vi "DataAcqMasterHD.vi"(0 "Avg Num":i32=1, 1 "2-D motor":bool, 2 "Type of scan":u16, 3 "Move motor":bool, 4 "Compile":bool, 5 "Therapy (T)":bool, 7 "Xmit Ring":i16, 9 "Current Plane":i32, 10 "lines per plane mod":i32, 11 "Total steps in line":i32, 12 "Acqiris ID":u32, 13 "Reverse ?":bool, 15 "CTR1":bool, 16 "start value":dbl, 17 "Motion System":u16, 18 "scan axis":i32, 19 "Motion Bd ID":T1 min=1 max=32 step=1) -> (20 "Samples Returned":i32, 21 "Motion error":bool, 22 "Timeout":bool, 23 "Raw VGain (scale)":dbl, 24 "Atts":dbl[](array[numeric]), 25 "Stacked Data":i16[][][](array[numeric]), 26 "error out":errorcluster)   [LabVIEW 2022 SP3]
uses:
  Motion Controllers/-MotionRoutines/MotionGlobals.vi
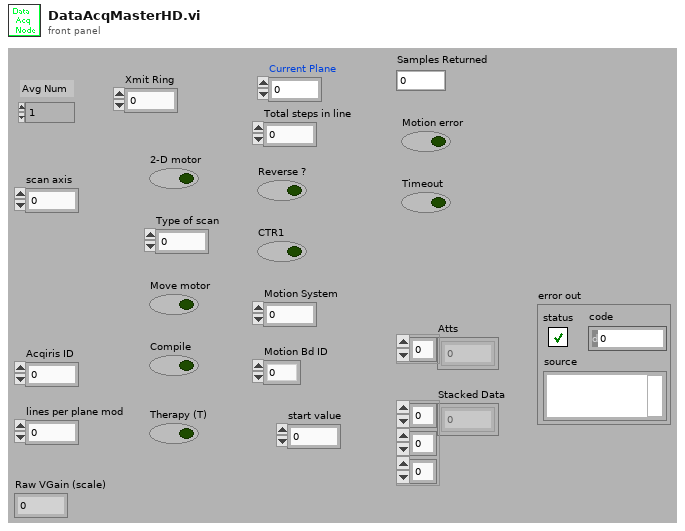
[diagram p1: front panel]
types:
  T1 = typedef "Board Id" = u8
  T2 = typedef "location.ctl" = enum16{"Automatic", "WCM Main", "Hawaii", "Columbia MM3000", "Columbia  NI System", "NYU", "RRI 2", "UHI Allen", "CUMC RT", "Chiba", "Stony Brook", "WCM Microscopy", "WCM Aeoretch", "WCM Optics Lab", "WCM Main 2Axis", "WCM Rotation", "WCM SAM SMAC", "SERI GP"}
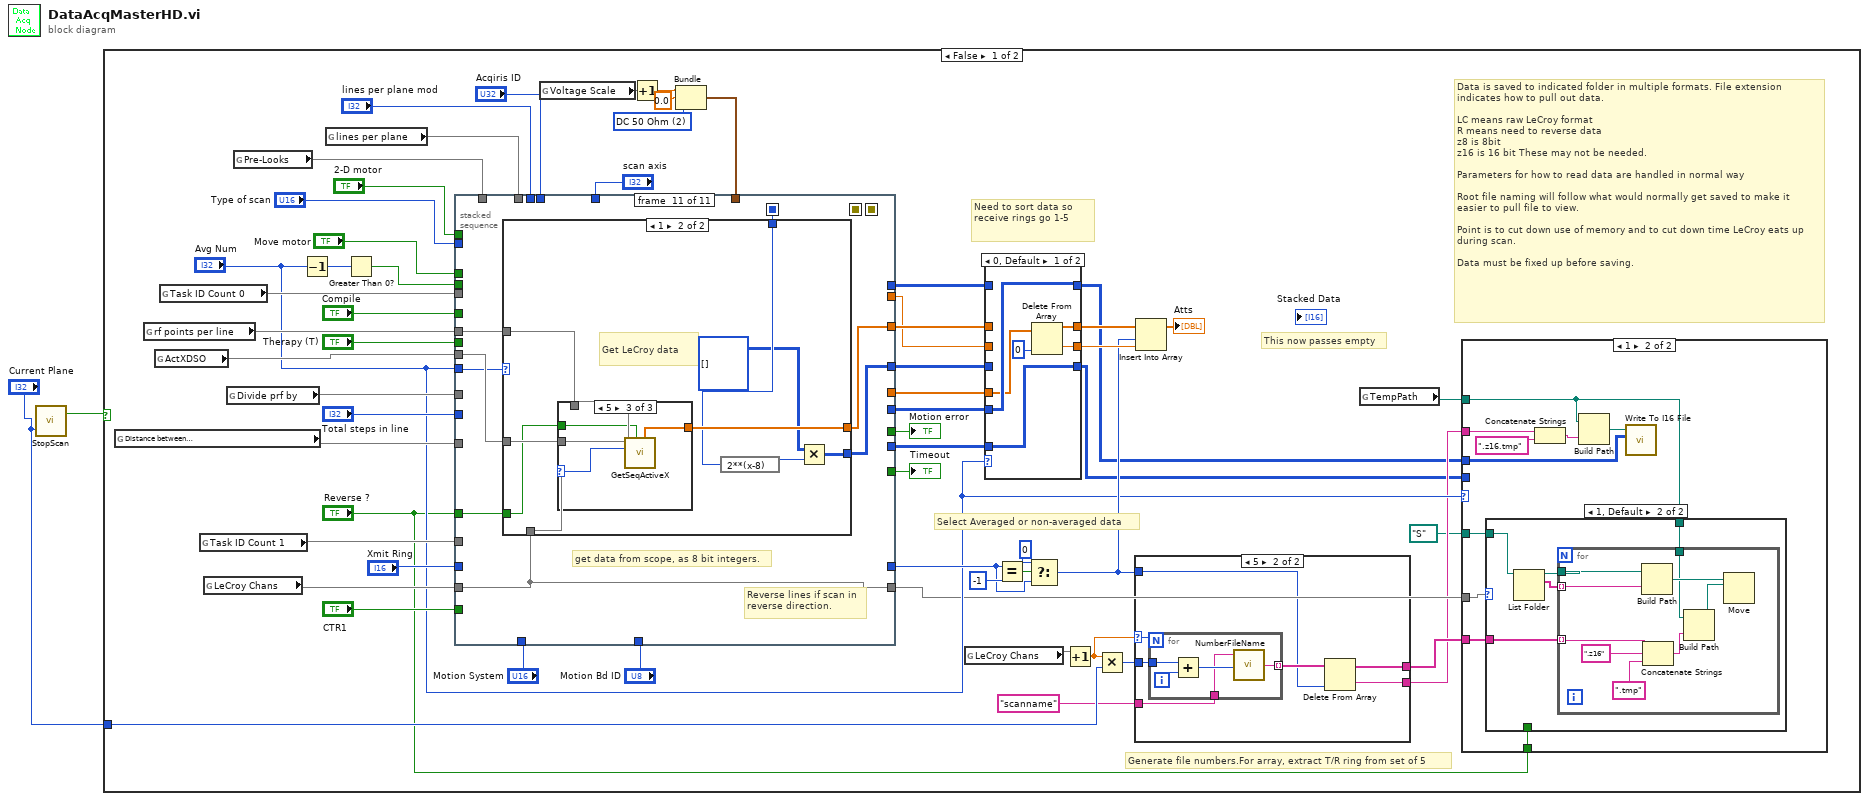
[diagram p0: block diagram]
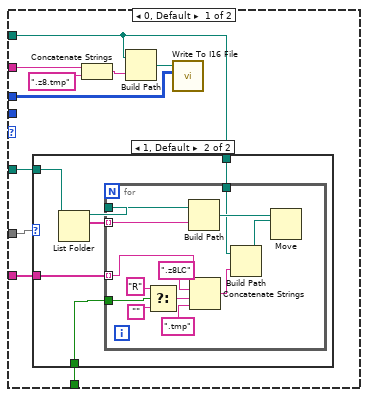
[diagram p2: hidden frame]
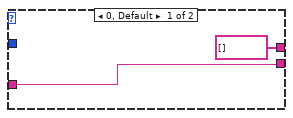
[diagram p5: hidden frame]
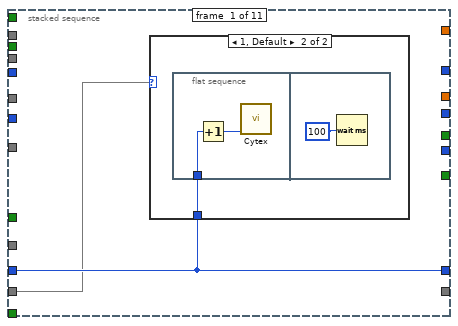
[diagram p7: hidden frame]
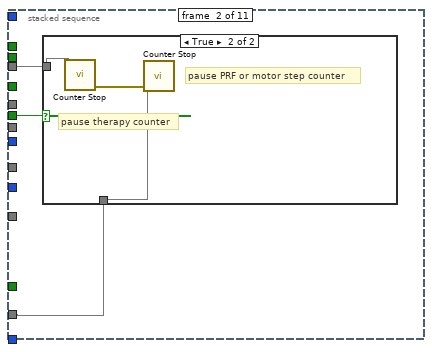
[diagram p9: hidden frame]
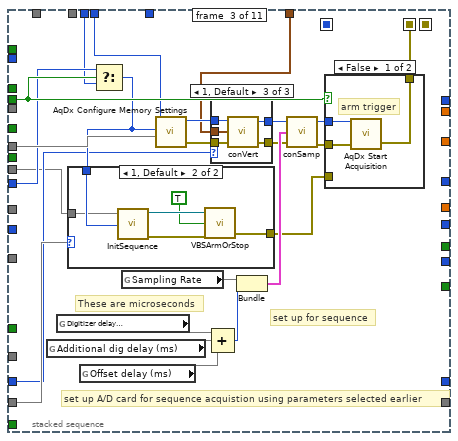
[diagram p11: hidden frame]
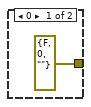
[diagram p15: hidden frame]
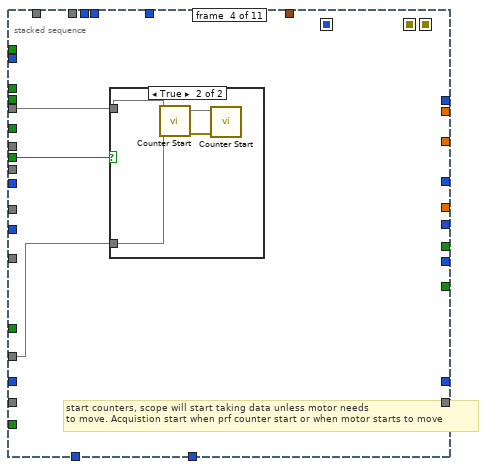
[diagram p16: hidden frame]
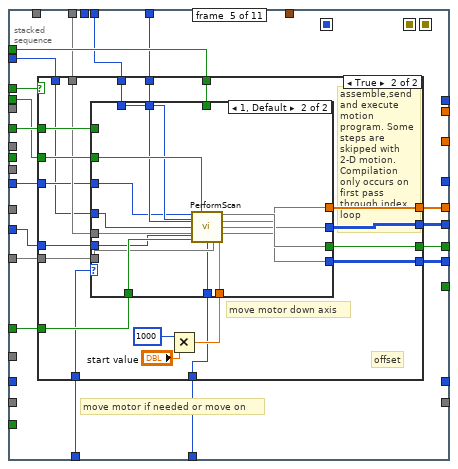
[diagram p18: hidden frame]
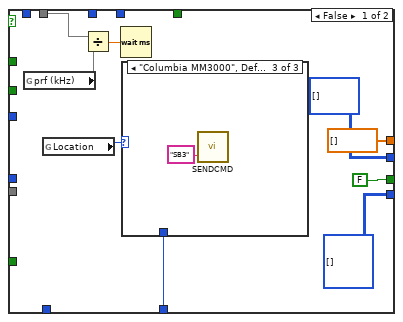
[diagram p19: hidden frame]
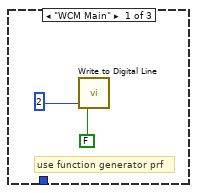
[diagram p20: hidden frame]
diagram:
  n1 = call "StopScan.vi"("Current Plane"="Current Plane") -> ("Stop Now? Dup"=w2:bool)  [unwired: 2 in]
  n2 = case shown="False" w2 {
    tunnel: "Current Plane" -> [w17 _]
    frame False {
      w24 = u16 2 items=["DC 1 MOhm", "AC 1 MOhm", "DC 50 Ohm", "AC 50 OHM"] ("Coupling")
      # "This now passes empty"
      # "Data is saved to indicated folder in multiple formats. File extension indicates how to pull out data.\n\nLC means raw LeCroy format\nR means need to reverse data\nz8 is 8bit\nz16 is 16 bit These may not be needed.\n\nParameters for how to read data are handled in normal way\n\nRoot file naming will follow what would normally get saved to make it easier to pull file to view.\n\nPoint is to cut down use of memory and to cut down time LeCroy eats up during scan.\n\nData must be fixed up before saving."
      # "Generate file numbers.For array, extract T/R ring from set of 5"
      # "Need to sort data so receive rings go 1-5"
      # "Select Averaged or non-averaged data"
      n3 = global read "MotionGlobals.vi" "Distance between\nscan lines (mm)"() -> (w49)
      n4 = global read "MotionGlobals.vi" "rf points per line"() -> (w48)
      n5 = global read "MotionGlobals.vi" "ActXDSO"() -> (w18)
      n6 = global read "MotionGlobals.vi" "Task ID Count 0"() -> (w22)
      n7 = global read "MotionGlobals.vi" "Task ID Count 1"() -> (w21)
      n8 = global read "MotionGlobals.vi" "LeCroy Chans"() -> (w44)
      n9 = global read "MotionGlobals.vi" "Divide prf by"() -> (w45)
      n10 = global read "MotionGlobals.vi" "Pre-Looks"() -> (w46)
      n11 = Decrement(x="Avg Num") -> (x-1=w19:i32)
      n12 = global read "MotionGlobals.vi" "lines per plane"() -> (w47)
      n13 = Greater Than 0?(x=w19) -> (x > 0?=w20:bool)
      n14 = global read "MotionGlobals.vi" "Voltage Scale"() -> (w25)
      n15 = Increment(x=w25) -> (x+1=w26:dbl)
      n16 = Bundle(w26, "Offset"=0.0, "Coupling"=w24) -> (w23:cluster{dbl, "Offset":dbl, "Coupling":u16})  [unwired: 1 in]
      n17 = stacked-sequence {
        seq-local: [_ _ w168 _ _ _ _ _ _ _ _] -> [_ _ _ _ _ w289 _ _ _ _ _]
        seq-local: [_ _ _ _ _ w287 _ _ _ _ _] -> [_ _ _ _ _ _ _ _ w340 _ _]
        seq-local: [_ _ _ _ _ _ _ _ w334 _ _] -> [_ _ _ _ _ _ _ _ _ _ w371]
        tunnel: "Therapy (T)" -> [_ w147 _ w196 _ _ w320 _ _ _ _]
        tunnel: w45 -> [_ _ _ _ _ _ _ _ w342 _ _]
        tunnel: "Move motor" -> [_ _ _ _ w219 _ _ w326 _ _ _]
        tunnel: "2-D motor" -> [_ _ _ _ w217 _ _ _ _ _ _]
        tunnel: "scan axis" -> [_ _ _ _ w213 _ _ _ _ _ _]
        tunnel: "Reverse ?" -> [_ _ _ _ w218 _ _ _ w338 _ w378]
        tunnel: "lines per plane mod" -> [_ _ w154 _ _ _ _ _ _ _ _]
        tunnel: "Total steps in line" -> [_ _ _ _ w215 _ _ _ _ _ _]
        tunnel: "Compile" -> [_ _ _ _ w216 _ _ _ _ _ _]
        tunnel: "CTR1" -> [_ _ _ _ _ _ _ _ _ _ _]
        tunnel: [_ _ _ _ _ w288 _ _ _ _ _] -> w57
        tunnel: "Acqiris ID" -> [_ _ w156 _ w208 w290 _ _ w339 _ _]
        tunnel: [_ _ _ _ _ _ _ _ w345 _ _] -> w42
        tunnel: "Type of scan" -> [_ _ _ _ w202 _ _ _ w344 _ _]
        tunnel: w47 -> [_ _ _ _ w214 w285 _ _ w343 _ _]
        tunnel: w46 -> [_ _ _ _ _ _ _ _ w341 _ _]
        tunnel: [_ _ _ _ w212 _ _ _ _ _ _] -> w60
        tunnel: "Motion System" -> [_ _ _ _ w211 _ _ _ _ _ _]
        tunnel: "Motion Bd ID" -> [_ _ _ _ w210 _ _ w325 _ _ _]
        tunnel: [_ _ _ _ _ _ _ _ _ _ w373] -> w40
        tunnel: w21 -> [_ w146 _ w197 _ _ w319 _ _ _ _]
        tunnel: w22 -> [_ w148 _ w198 _ _ w321 _ _ _ _]
        tunnel: w18 -> [_ _ w153 _ _ _ _ _ _ w365 w377]
        tunnel: w49 -> [_ _ _ _ w209 _ _ _ _ _ _]
        tunnel: w44 -> [w140 _ w163 _ _ _ _ _ _ w363 w374]
        tunnel: w48 -> [_ _ w165 _ _ _ _ _ w337 _ w376]
        tunnel: w20 -> [_ _ w166 _ w207 _ _ _ _ _ _]
        tunnel: "Avg Num" -> [_ _ w155 _ w206 w286 _ _ w336 w364 w375]
        tunnel: [_ _ _ _ w205 _ _ _ _ _ _] -> w39
        tunnel: [_ _ _ _ w204 _ _ _ _ _ _] -> w37
        tunnel: [_ _ _ _ w203 _ _ _ _ _ _] -> w38
        tunnel: [_ _ _ _ _ _ _ _ _ _ w372] -> w41
        tunnel: [w141 _ _ _ _ _ _ _ _ _ _] -> w29
        tunnel: "Xmit Ring" -> [w141 _ w158 _ _ _ _ _ _ _ _]
        tunnel: [_ _ _ _ _ _ _ _ w335 _ _] -> w32
        tunnel: w23 -> [_ _ w157 _ _ _ _ _ _ _ _]
        tunnel: [_ _ _ _ _ _ _ _ _ _ w374] -> w10
        frame #0 {
          n18 = case shown="1, Default" w140 {
            tunnel: w141 -> [_ w142]
            frame 0 {
            }
            frame 1, Default {
              n19 = flat-sequence {
                tunnel: w142 -> [w144]
                frame #0 {
                  n20 = Increment(x=w144) -> (x+1=w143:i16)
                  n21 = call "Cytex.vi"("Xmit Ring"=w143) -> ()  [unwired: 1 in, 2 out]
                }
                frame #1 {
                  n22 = Wait (ms)(milliseconds to wait=100) -> ()  [unwired: 1 out]
                }
              }
            }
          }
        }
        frame #1 {
          n23 = case shown="True" w147 {
            tunnel: w148 -> [_ w151]
            tunnel: w146 -> [_ w149]
            frame False {
            }
            frame True {
              # "pause PRF or motor step counter"
              # "pause therapy counter"
              n24 = call <vilib>:"Counter Stop.vi"("taskID"=w151) -> ("error out"=w150:errorcluster)  [unwired: 5 in, 1 out]
              n25 = call <vilib>:"Counter Stop.vi"("error in (no error)"=w150, "taskID"=w149) -> ()  [unwired: 4 in, 2 out]
            }
          }
        }
        frame #2 {
          # "These are microseconds"
          # "set up for sequence"
          # "set up A/D card for sequence acquistion using parameters selected earlier"
          n26 = global read "MotionGlobals.vi" "Additional dig delay (ms)"() -> (w171)
          n27 = global read "MotionGlobals.vi" "Digitizer delay\n (ms)"() -> (w174)
          n28 = global read "MotionGlobals.vi" "Offset delay (ms)"() -> (w167)
          n29 = Select(t=w155, s=w166, f=w154) -> (s? t:f=w164:i32)
          n30 = case shown="1, Default" w163 {
            tunnel: w164 -> [_ w195]
            tunnel: w153 -> [_ w194]
            tunnel: [errorcluster {"status"=FALSE, "code"=0, "source"=""} ("error out") w190] -> w152
            frame 0 {
            }
            frame 1, Default {
              n31 = call "InitSequence.vi"("ActXDSO In"=w194, "Num of Sequences"=w195) -> ("ActXDSO Out"=w193:refnum<k7>, "error out"=w192:errorcluster)  [unwired: 5 in]
              n32 = call "VBSArmOrStop.vi"("error in (no error)"=w192, "Arm T/Stop F"=TRUE, "ActXDSO In"=w193) -> ("error out"=w190:errorcluster)  [unwired: 1 in, 1 out]
            }
          }
          n33 = global read "MotionGlobals.vi" "Sampling Rate"() -> (w173)
          n34 = call "AqDx Configure Memory Settings.vi"("Number of Samples (1000)"=w165, "Number of Segments (1)"=w164, "Instrument ID"=w156) -> ("error out"=w159:errorcluster, "dup Instrument ID"=w160:u32)  [unwired: 3 in]
          n35 = case shown="1, Default" w158 {
            tunnel: [w177 w179 w184] -> w162
            tunnel: [w176 w178 w183] -> w161
            tunnel: w160 -> [w177 w179 w182]
            tunnel: w159 -> [w176 w178 w181]
            tunnel: w157 -> [_ _ w180]
            frame 0 {
            }
            frame -1 {
            }
            frame 1, Default {
              n36 = call "conVert.vi"("InstrumentID"=w182, "V scale"=w180, "error in"=w181) -> ("Status"=w184:i32, "error out"=w183:errorcluster)  [unwired: 3 in]
            }
          }
          n37 = Compound Arithmetic op=ADD(w174, w171, w167) -> (w172:i32)
          n38 = Bundle("Sampling Rate"=w173, w172) -> (w175:cluster{"Sampling Rate":void, i32})  [unwired: 1 in]
          n39 = call "conSamp.vi"("error in"=w161, "Sampling"=w175, "InstrumentID"=w162) -> ("error out"=w169:errorcluster, "DUP ID"=w170:u32)
          n40 = case shown="False" w166 {
            tunnel: w170 -> [w187 _]
            tunnel: w169 -> [w186 w188]
            tunnel: [w185 w188] -> w168
            tunnel: w152 -> [_ _]
            frame False {
              # "arm trigger"
              n41 = call "AqDx Start Acquisition.vi"("error in (no error)"=w186, "Instrument ID"=w187) -> ("error out"=w185:errorcluster)  [unwired: 1 in, 1 out]
            }
            frame True {
            }
          }
        }
        frame #3 {
          # "start counters, scope will start taking data unless motor needs\nto move. Acquistion start when prf counter start or when motor starts to move"
          n42 = case shown="True" w196 {
            tunnel: w198 -> [_ w201]
            tunnel: w197 -> [_ w199]
            frame False {
            }
            frame True {
              n43 = call <vilib>:"Counter Start.vi"("taskID"=w201) -> ("error out"=w200:errorcluster)  [unwired: 9 in, 1 out]
              n44 = call <vilib>:"Counter Start.vi"("error in (no error)"=w200, "taskID"=w199) -> ()  [unwired: 8 in, 2 out]
            }
          }
        }
        frame #4 {
          # "move motor if needed or move on"
          n45 = case shown="True" w219 {
            tunnel: w209 -> [_ w251]
            tunnel: w218 -> [_ w253]
            tunnel: w207 -> [_ w252]
            tunnel: w217 -> [_ w250]
            tunnel: w216 -> [_ w249]
            tunnel: w215 -> [_ w248]
            tunnel: w214 -> [w221 w244]
            tunnel: w213 -> [_ w247]
            tunnel: [FALSE w246] -> w212
            tunnel: w211 -> [_ w245]
            tunnel: w210 -> [w226 w235]
            tunnel: w208 -> [_ w243]
            tunnel: w206 -> [_ w242]
            tunnel: [dbl[] [] ("Att (dB)") w241] -> w205
            tunnel: [i16[][] [] ("Acqiris Avg") w240] -> w204
            tunnel: [i16[][][] [] ("Acqiris Avg") w239] -> w203
            tunnel: w202 -> [_ w234]
            frame False {
              n46 = global read "MotionGlobals.vi" "prf (kHz)"() -> (w220)
              n47 = global read "MotionGlobals.vi" "Location"() -> (w227:T2)
              n48 = Divide(x=w221, y=w220) -> (x/y=w222:dbl)
              n49 = Wait (ms)(milliseconds to wait=w222) -> ()  [unwired: 1 out]
              n50 = case shown="\"Columbia MM3000\", Default" w227 {
                tunnel: w226 -> [_ w231 _]
                frame "WCM Main" {
                  # "use function generator prf"
                  n51 = call <vilib>:"Write to Digital Line.vi"("line"=2, "line state"=FALSE) -> ()  [unwired: 7 in]
                }
                frame "Hawaii" {
                  # "Use BreakPt PRF"
                  n52 = call <vilib>:"Run Program.flx"("Program (1)"=3, "Board ID"=w231) -> ()  [unwired: 4 in, 3 out]
                }
                frame "Columbia MM3000", Default {
                  n53 = call "SENDCMD.VI"("MM2000 Command (ASCII String)"="SB3") -> ()  [unwired: 2 in, 1 out]
                }
              }
            }
            frame True {
              # "assemble,send and execute\nmotion program. Some steps are\nskipped with 2-D motion. Compilation only occurs on first pass through index loop"
              # "offset"
              # "move motor down axis"
              n54 = Multiply(x=1000, y="start value") -> (x*y=w236:dbl)
              n55 = case shown="1, Default" w245 {
                tunnel: w253 -> [w269 w284]
                tunnel: w252 -> [w268 w283]
                tunnel: w251 -> [w267 w282]
                tunnel: w250 -> [w266 _]
                tunnel: w249 -> [w265 _]
                tunnel: w248 -> [w264 w281]
                tunnel: w247 -> [w263 w280]
                tunnel: [w256 w276] -> w246
                tunnel: w244 -> [w262 w279]
                tunnel: w243 -> [w261 w278]
                tunnel: w242 -> [w260 w277]
                tunnel: [w259 w273] -> w241
                tunnel: [w258 w274] -> w240
                tunnel: [w257 w275] -> w239
                tunnel: w236 -> [w255 w272]
                tunnel: w235 -> [_ w271]
                tunnel: w234 -> [w254 w270]
                frame 0 {
                  n56 = call "SendProgram.vi"("Type of scan"=w254, "Line Axis"=w263, "Avg Num"=w260, "lines per scan plane"=w262, "Reverse ?"=w269, "Therapy/AVG ?"=w268, 7:w264, 8:w261, 12:w266, 13:w267, 14:w265, "Offset"=w255) -> ("Error Status"=w256:bool, 16:w259, 17:w258, 18:w257)  [unwired: 4 in]
                }
                frame 1, Default {
                  n57 = call "PerformScan.vi"("Avg Num Mod"=w277, "Therapy/AVG ?"=w283, "AlazarCluster"=w278, "Line Axis"=w280, "Type of scan"=w270, "lines per scan plane mod"=w279, "Reverse ?"=w284, "Digitizer Settings"=w281, "Motion Settings In"=w271, "File Names"=w282, "Offset"=w272) -> (4:w276, 6:w273, 8:w274, 10:w275)  [unwired: 1 in]
                }
              }
            }
          }
        }
        frame #5 {
          n58 = case shown="1" w286 {
            tunnel: w290 -> [_ w298]
            tunnel: w289 -> [w292 w299]
            tunnel: [FALSE w297] -> w288
            tunnel: [w292 w295] -> w287
            tunnel: w285 -> [_ w296]
            frame 0, Default {
            }
            frame 1 {
              # "Check to see if data acquistion is finished. WaitTWO seconds\nmore and then force extra trigs if needed. Data should all be taken be the time this frame is reached. May need more sophisticated error checking"
              n59 = call "AqDx Wait For End Of Acquisition.vi"("error in (no error)"=w299, "Timeout"=2000, "Instrument ID"=w298) -> ("error out"=w294:errorcluster, "dup Instrument ID"=w293:u32)  [unwired: 3 in]
              n60 = Unbundle(w294) -> ("status"=w297:bool)  [unwired: 2 out]
              n61 = case shown="True" w297 {
                tunnel: w294 -> [w301 _]
                tunnel: w293 -> [w302 w310]
                tunnel: w296 -> [_ w309]
                tunnel: [w301 w303] -> w295
                tunnel: [w302 w304] -> _
                frame False {
                }
                frame True {
                  n62 = call "AqDx Query Number of Acquired Segments.vi"("Instrument ID"=w310) -> ("error out"=w305:errorcluster, "Number of Segments"=w308:i32, "dup Instrument ID"=w306:u32)  [unwired: 4 in]
                  n63 = Subtract(x=w309, y=w308) -> (x-y=w307:i32)
                  n64 = for {
                    N: w307 -> [_]
                    tunnel: w305 -> [w318]
                    tunnel: w306 -> [w317]
                    tunnel: [w314] -> w304
                    tunnel: [w313] -> w303
                    n65 = call "AqDx Software Trigger.vi"("error in (no error)"=w318, "Type"=1, "Instrument ID"=w317) -> ("error out"=w315:errorcluster, "dup Instrument ID"=w312:u32)
                    n66 = call "AqDx Wait For End Of Acquisition.vi"("error in (no error)"=w315, "Timeout"=3, "Instrument ID"=w312) -> ("error out"=w313:errorcluster, "dup Instrument ID"=w314:u32)  [unwired: 3 in]
                  }
                }
              }
            }
          }
        }
        frame #6 {
          n67 = case shown="True" w320 {
            tunnel: w321 -> [_ w324]
            tunnel: w319 -> [_ w322]
            frame False {
            }
            frame True {
              # "stop counters again"
              # "stop therapy counter"
              n68 = call <vilib>:"Counter Stop.vi"("taskID"=w324) -> ("error out"=w323:errorcluster)  [unwired: 5 in, 1 out]
              n69 = call <vilib>:"Counter Stop.vi"("error in (no error)"=w323, "taskID"=w322) -> ()  [unwired: 4 in, 2 out]
            }
          }
        }
        frame #7 {
          # "turn off function generator prf"
          n70 = case shown="False" w326 {
            tunnel: w325 -> [w327 _]
            frame False {
              n71 = global read "MotionGlobals.vi" "Location"() -> (w328:T2)
              n72 = case shown="\"Columbia MM3000\", Default" w328 {
                tunnel: w327 -> [_ w331 _]
                frame "WCM Main" {
                  n73 = call <vilib>:"Write to Digital Line.vi"("line"=2, "line state"=TRUE) -> ()  [unwired: 7 in]
                }
                frame "Hawaii" {
                  n74 = call <vilib>:"Stop Program.flx"("Program (1)"=3, "Board ID"=w331) -> ()  [unwired: 4 in, 3 out]
                }
                frame "Columbia MM3000", Default {
                  n75 = call "SENDCMD.VI"("MM2000 Command (ASCII String)"="CB3") -> ()  [unwired: 2 in, 1 out]
                }
              }
            }
            frame True {
            }
          }
        }
        frame #8 {
          # "Reverse lines if scan in \nreverse direction."
          # "get data from scope, as 8 bit integers."
          n76 = case shown="1" w336 {
            tunnel: [i16[][] [] ("Array") w362] -> w345
            tunnel: w344 -> [_ w361]
            tunnel: w343 -> [_ w360]
            tunnel: w342 -> [_ w359]
            tunnel: w341 -> [_ w358]
            tunnel: w340 -> [_ w357]
            tunnel: w339 -> [_ w356]
            tunnel: w338 -> [_ w351]
            tunnel: w337 -> [_ w354]
            tunnel: [0.0 w352] -> w335
            tunnel: [8 w349] -> w334
            frame 0, Default {
            }
            frame 1 {
              # "Might need to scale LeCroy data"
              n77 = call "GetAcqSeq.vi"("Pre-Looks"=w358, "lines per plane"=w360, "Acqiris ID"=w356, "Type of scan"=w361, "rf points per line"=w354, "errorin"=w357, "Divide prf by"=w359, "Reverse?"=w351) -> ("Array"=w362:i16[][], "VGain (dB)"=w352:dbl, "Dig Word Size"=w349:u16, "returnedSamplesPerSeg"=→"Samples Returned":i32, "Raw VGain (scale)"=→"Raw VGain (scale)":dbl, "error out"=→"error out":errorcluster)  [unwired: 1 in, 1 out]
              n78 = global write "MotionGlobals.vi" "bits A/D"(w349) -> ()
            }
          }
        }
        frame #9 {
          n79 = case shown="1" w364 {
            tunnel: w365 -> [_ w367]
            tunnel: w363 -> [_ w366]
            frame 0, Default {
              (unwired) FALSE
            }
            frame 1 {
              # "Check to see if data acquistion is finished. WaitTWO seconds\nmore and then force extra trigs if needed. Data should all be taken be the time this frame is reached. May need more sophisticated error checking.THis is done after get acqirs data because the LeCroy is slower. Might buy some time here."
              n80 = case shown="1, Default" w366 {
                tunnel: w367 -> [w368 w370]
                tunnel: [w368 w369] -> _
                frame 0 {
                }
                frame 1, Default {
                  n81 = call "AcqWait.vi"("ActXDSO In"=w370) -> ("ActXDSO Out"=w369:refnum<k7>)  [unwired: 1 in, 1 out]
                }
              }
            }
          }
        }
        frame #10 {
          # "Reverse lines if scan in \nreverse direction."
          # "get data from scope, as 8 bit integers."
          n82 = case shown="1" w375 {
            tunnel: [i16[][][] [] ("Data") w387] -> w373
            tunnel: w378 -> [_ w383]
            tunnel: w377 -> [_ w389]
            tunnel: w376 -> [_ w388]
            tunnel: [dbl[] [] w385] -> w372
            tunnel: w374 -> [_ w384]
            tunnel: w371 -> [_ w382]
            frame 0, Default {
            }
            frame 1 {
              # "Get LeCroy data"
              n83 = case shown="5" w384 {
                selector: w384 -> [_ w392 w395]
                tunnel: w389 -> [_ w391 w394]
                tunnel: w388 -> [_ _ w398]
                tunnel: w383 -> [_ _ w397]
                tunnel: [dbl[] [] ("Att (dB)") w393 w396] -> w385
                frame 0 {
                }
                frame 1, Default {
                  n84 = call "GetSavedTCP.vi"("Channels to Acq"=w392, "ActiveDSO In"=w391) -> ("Att (dB)"=w393:dbl[])  [unwired: 6 in, 3 out]
                }
                frame 5 {
                  n85 = call "GetSeqActiveX.vi"("Reverse?"=w397, "RF Points"=w398, "Channels to Acq"=w395, "ActiveDSO In"=w394) -> ("Att (dB)"=w396:dbl[])  [unwired: 3 in, 4 out]
                }
              }
              n86 = expression code="2**(x-8)"(w382) -> (w386:i32)
              n87 = Multiply(x=i16[][][] [] ("Data"), y=w386) -> (x*y=w387:i32[][][])
            }
          }
        }
      }
      "Motion error" <- w60
      "Timeout" <- w57
      n88 = global read "MotionGlobals.vi" "LeCroy Chans"() -> (w15)
      n89 = case shown="0, Default" "Avg Num" {
        tunnel: [w134 w139] -> w6
        tunnel: w42 -> [_ w139]
        tunnel: w41 -> [_ w138]
        tunnel: [w132 w138] -> w34
        tunnel: w40 -> [_ w137]
        tunnel: [w135 w137] -> w5
        tunnel: w39 -> [w133 _]
        tunnel: w38 -> [w135 _]
        tunnel: w37 -> [w134 _]
        tunnel: [w131 w136] -> w33
        tunnel: w32 -> [_ w136]
        frame 0, Default {
          n90 = Delete From Array(array=w133, index=0) -> (deleted portion=w131:dbl, array with subset deleted=w132:dbl[])  [unwired: 1 in]
        }
        frame 1 {
        }
      }
      n91 = Equal?(x=w29, y=-1) -> (x = y?=w31:bool)
      n92 = Select(t=0, s=w31, f=w29) -> (s? t:f=w12:i32)
      n93 = Increment(x=w15) -> (x+1=w14:dbl)
      n94 = Multiply(x=w14, y=w17) -> (x*y=w16:i32)
      n95 = case shown="5" w14 {
        selector: w14 -> [_ w118]
        tunnel: w16 -> [_ w124]
        tunnel: "scanname" -> [w116 w123]
        tunnel: w12 -> [_ w121]
        tunnel: [w116 w120] -> w8
        tunnel: [string[] [] w119] -> w9
        frame 0, Default {
        }
        frame 5 {
          n96 = for {
            N: w118 -> [_]
            tunnel: w124 -> [w128]
            tunnel: w123 -> [w126]
            tunnel: [w125] -> w122 mode=indexing
            i -> [w129]
            n97 = Add(x=w128, y=w129) -> (x+y=w127:i32)
            n98 = call "NumberFileName.vi"("File number"=w127, "file name"=w126) -> ("Numbered File"=w125:string)  [unwired: 1 in]
          }
          n99 = Delete From Array(array=w122, index=w121) -> (deleted portion=w120:string, array with subset deleted=w119:string[])  [unwired: 1 in]
        }
      }
      n100 = Insert Into Array(array=w34, index=w12, new element=w33) -> (→"Atts":dbl[])
      n101 = global read "MotionGlobals.vi" "TempPath"() -> (w3:path)
      n102 = case shown="1" "Avg Num" {
        tunnel: w10 -> [w72 w101]
        tunnel: w9 -> [w71 w100]
        tunnel: w8 -> [w69 w98]
        tunnel: "Reverse ?" -> [w68 w97]
        tunnel: w6 -> [w67 w96]
        tunnel: w3 -> [w64 w93]
        tunnel: w5 -> [_ _]
        tunnel: path "S:/" ("file path (dialog if empty)") -> [w63 w92]
        frame 0, Default {
          n103 = case shown="1, Default" w72 {
            tunnel: w71 -> [_ w76]
            tunnel: w68 -> [_ w75]
            tunnel: w64 -> [_ w74]
            tunnel: w63 -> [_ w73]
            frame 0 {
            }
            frame 1, Default {
              n104 = List Folder(path=w73) -> (path out=w77:path, filenames=w78:string[])  [unwired: 3 in, 2 out]
              n105 = for {
                tunnel: w78 -> [w91] mode=indexing
                tunnel: w77 -> [w90]
                tunnel: w76 -> [w82] mode=indexing
                tunnel: w75 -> [w80]
                tunnel: w74 -> [w79]
                n106 = Select(t="R", s=w80, f="") -> (s? t:f=w86:string)
                n107 = Build Path(base path=w90, name or relative path=w91) -> (appended path=w89:path)
                n108 = Concatenate Strings(w82, ".z8LC", w86, ".tmp") -> (w83:string)
                n109 = Build Path(base path=w79, name or relative path=w83) -> (appended path=w85:path)
                n110 = Move(source path=w89, 10:w85) -> ()  [unwired: 3 in, 3 out]
              }
            }
          }
          n111 = Concatenate Strings(w69, ".z8.tmp") -> (w65:string)
          n112 = Build Path(base path=w64, name or relative path=w65) -> (appended path=w66:path)
          n113 = call <vilib>:"Write To I16 File.vi"("2D array"=w67, "file path (dialog if empty)"=w66) -> ()  [unwired: 5 in, 1 out]
        }
        frame 1 {
          n114 = case shown="1, Default" w101 {
            tunnel: w100 -> [_ w104]
            tunnel: w97 -> [_ _]
            tunnel: w93 -> [_ w103]
            tunnel: w92 -> [_ w102]
            frame 0 {
            }
            frame 1, Default {
              n115 = List Folder(path=w102) -> (path out=w105:path, filenames=w106:string[])  [unwired: 3 in, 2 out]
              n116 = for {
                tunnel: w106 -> [w115] mode=indexing
                tunnel: w105 -> [w114]
                tunnel: w104 -> [w109] mode=indexing
                tunnel: w103 -> [w107]
                n117 = Build Path(base path=w114, name or relative path=w115) -> (appended path=w113:path)
                n118 = Concatenate Strings(w109, ".z16", ".tmp") -> (w110:string)
                n119 = Build Path(base path=w107, name or relative path=w110) -> (appended path=w111:path)
                n120 = Move(source path=w113, 10:w111) -> ()  [unwired: 3 in, 3 out]
              }
            }
          }
          n121 = Concatenate Strings(w98, ".z16.tmp") -> (w94:string)
          n122 = Build Path(base path=w93, name or relative path=w94) -> (appended path=w95:path)
          n123 = call <vilib>:"Write To I16 File.vi"("2D array"=w96, "file path (dialog if empty)"=w95) -> ()  [unwired: 5 in, 1 out]
        }
      }
    }
    frame True {
    }
  }
